vi "Create CSV with header.vi"(1 "Declared directory":path, 2 "Declare directory, else VI working directory is used for base file path":bool, 4 "CSV Header":string[][](array[string]), 5 "Folder name":string, 6 "error in":errorcluster, 7 "Trial #":i32, 8 "Append date to folder name":bool, 9 "File name":string) -> (0 "error out":errorcluster, 3 "File path":path)   [LabVIEW 2018]
uses:
  <vilib>/Utility/file.llb/Write Delimited Spreadsheet (string).vi
panel:
  out "Save path (folder)":path
  # "INPUTS"
  # "OUTPUTS"
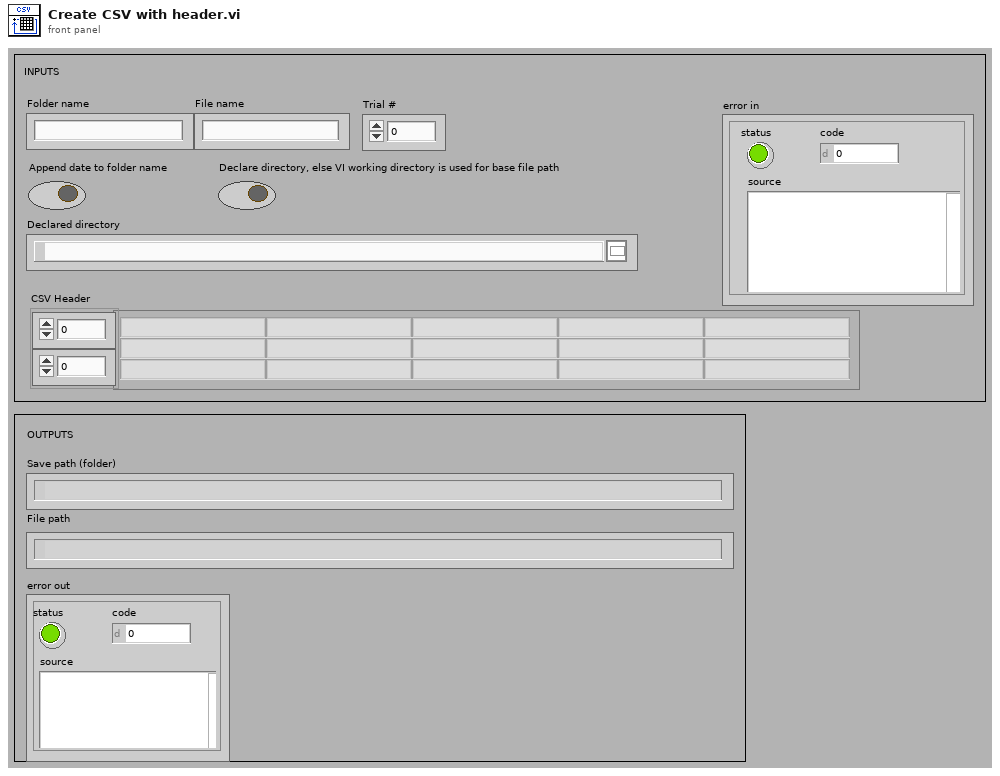
[diagram p1: front panel]
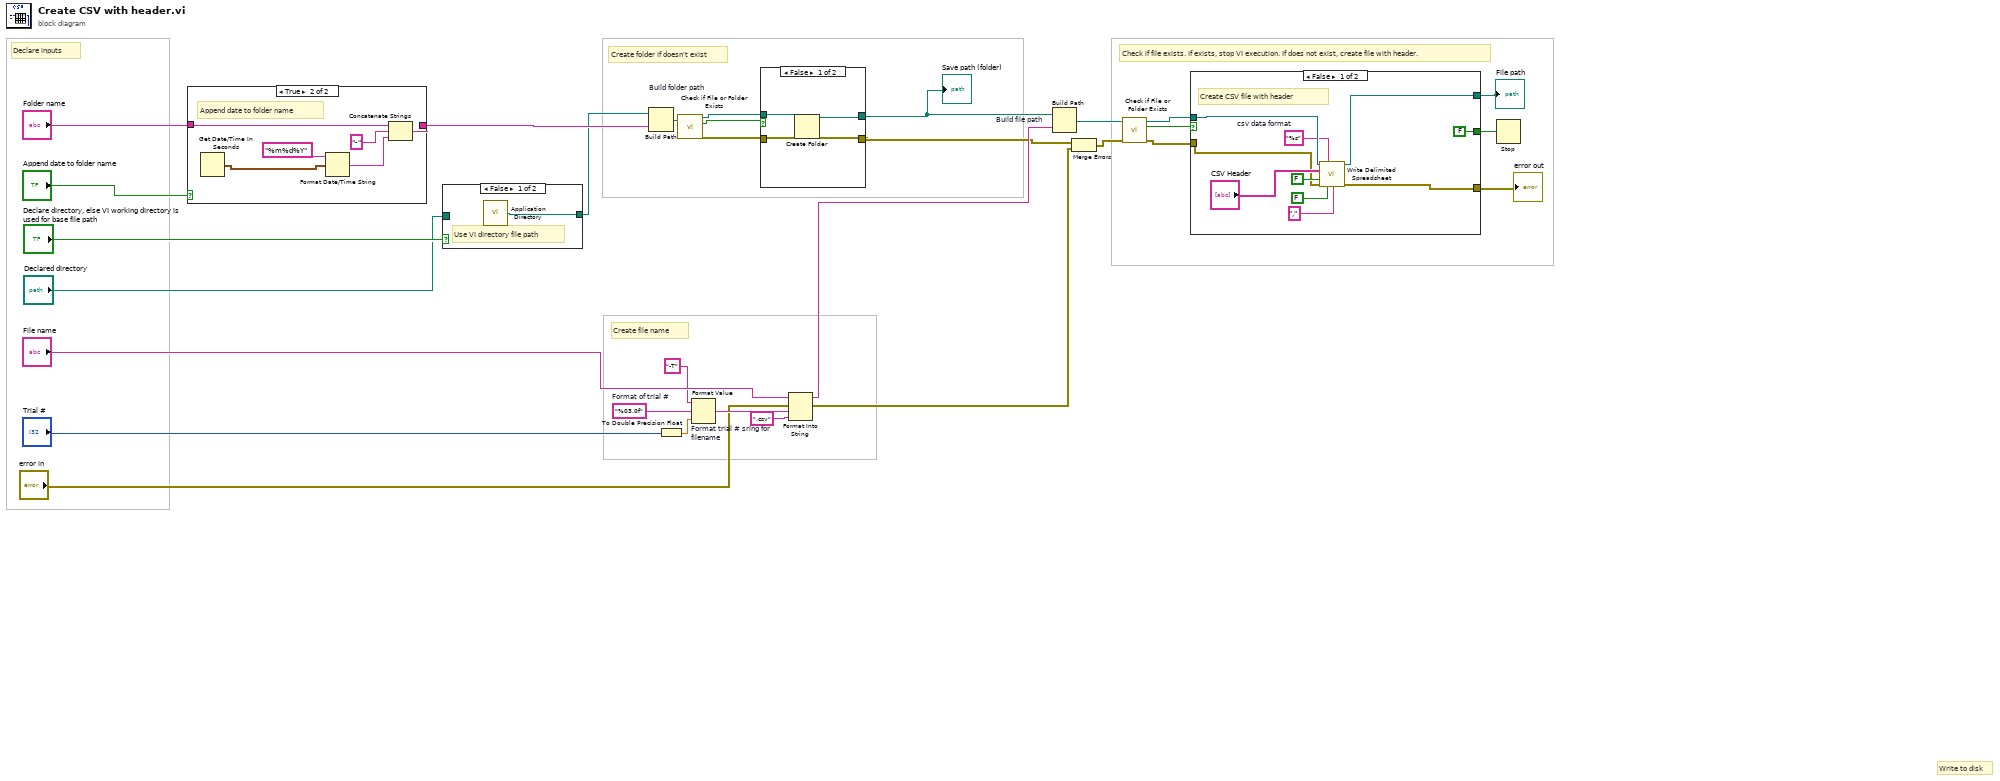
[diagram p0: block diagram]
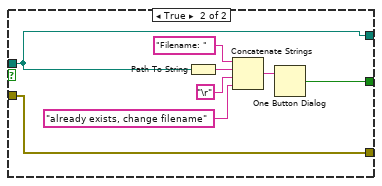
[diagram p4: hidden frame]
diagram:
  w23 = "%03.0f"  # Format of trial #
  # "Check if file exists. If exists, stop VI execution. If does not exist, create file with header."
  # "Create file name"
  # "Declare inputs"
  # "Create folder if doesn't exist"
  # "Write to disk"
  n1 = case shown="True" "Append date to folder name" {
    tunnel: "Folder name" -> [w31 w37]
    tunnel: [w31 w35] -> w8
    frame False {
    }
    frame True {
      # "Append date to folder name"
      n2 = Get Date/Time In Seconds() -> (seconds since 1Jan1904=w34:timestamp)
      n3 = Format Date/Time String(time format string (%c)="%m%d%Y", seconds (now)=w34) -> (date/time string=w32:string)  [unwired: 1 in]
      n4 = Concatenate Strings(w37, "-" ("string"), w32) -> (w35:string)
    }
  }
  n5 = case shown="False" "Declare directory, else VI working directory is used for base file path" {
    tunnel: [w38 w39] -> w7
    tunnel: "Declared directory" -> [_ w39]
    frame False {
      # "Use VI directory file path"
      n6 = call <vilib>:"Application Directory.vi"() -> ("Application Directory"=w38:path)
    }
    frame True {
      # "Use absolute file path"
    }
  }
  n7 = Build Path "Build folder path"(base path=w7, name or relative path=w8) -> (appended path=w27:path)
  n8 = To Double Precision Float(number="Trial #") -> (double precision float=w20:dbl)
  n9 = call <vilib>:"Check if File or Folder Exists.vi"("path"=w27) -> ("error out"=w30:errorcluster, "file or folder exists?"=w29:bool, "dup path"=w28:path)  [unwired: 8 in]
  n10 = Format Value "Format trial # sring for filename"(string ("")="-T" ("input 1"), format string=w23, value (0)=w20) -> (output string=w18:string)
  n11 = case shown="False" w29 {
    tunnel: w30 -> [w43 w44]
    tunnel: w28 -> [w42 w45]
    tunnel: [w41 w45] -> w26
    tunnel: [w40 w44] -> w2
    frame False {
      n12 = Create Folder(path (use dialog)=w42, error in=w43) -> (created path=w41:path, error out=w40:errorcluster)  [unwired: 1 in, 1 out]
    }
    frame True {
    }
  }
  "Save path (folder)" <- w26
  n13 = Format Into String "Format Into String"(initial string="File name", error in="error in", w18, ".csv" ("name or relative path")) -> (resulting string=w24:string, error out=w3:errorcluster)  [unwired: 1 in]
  n14 = Build Path "Build file path"(base path=w26, name or relative path=w24) -> (appended path=w17:path)
  n15 = Merge Errors(w2, w3) -> (w1:errorcluster)
  n16 = call <vilib>:"Check if File or Folder Exists.vi"("error in (no error)"=w1, "path"=w17) -> ("error out"=w15:errorcluster, "file or folder exists?"=w16:bool, "dup path"=w14:path)  [unwired: 7 in]
  n17 = case shown="False" w16 {
    tunnel: w15 -> [w50 w56]
    tunnel: w14 -> [w53 w57]
    tunnel: [FALSE w58] -> w13
    tunnel: [w47 w56] -> w5
    tunnel: [w46 w57] -> w12
    frame False {
      w52 = "%s"  # csv data format
      # "Create CSV file with header"
      n18 = call-poly <vilib>:"Write Delimited Spreadsheet.vi"("file path (dialog if empty)"=w53, "format (%s)"=w52, "2D data"="CSV Header", "append to file? (new file:F)"=FALSE, "error in (no error)"=w50, "transpose? (no:F)"=FALSE, "delimiter (\\t)"="," ("delimiter (\\t)")) -> ("new file path (Not A Path if cancelled)"=w46:path, "error out"=w47:errorcluster)  [unwired: 7 in]
    }
    frame True {
      n19 = Path To String(path=w57) -> (string=w61:string)
      n20 = Concatenate Strings("Filename: " ("string"), w61, "\r", "already exists, change filename" ("string")) -> (w63:string)
      n21 = One Button Dialog(message=w63) -> (true=w58:bool)  [unwired: 1 in]
    }
  }
  "File path" <- w12
  "error out" <- w5
  n22 = Stop(stop? (T)=w13) -> ()
